vi "Set Line.vi"(8 "error in (no error)":errorcluster, 10 "First Visible Line":i32, 11 "ScintillaNET in":refnum<class "ScintillaNET.lvclass">) -> (0 "error out":errorcluster, 3 "ScintillaNET out":refnum<class "ScintillaNET.lvclass">)   [LabVIEW 2018, in "ScintillaNET.lvclass"]
uses:
  ScintillaNET.lvclass
  ScintillaNET.lvclass/ScintillaNET.ctl
  D:/project/hobby/LF2R/LabVIEW/source/ScintillaNET/dll/ScintillaNET.dll
  dll/ScintillaNET.dll
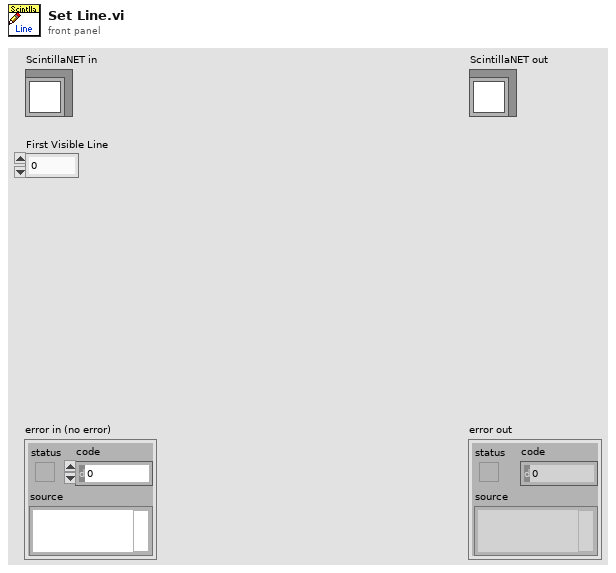
[diagram p1: front panel]
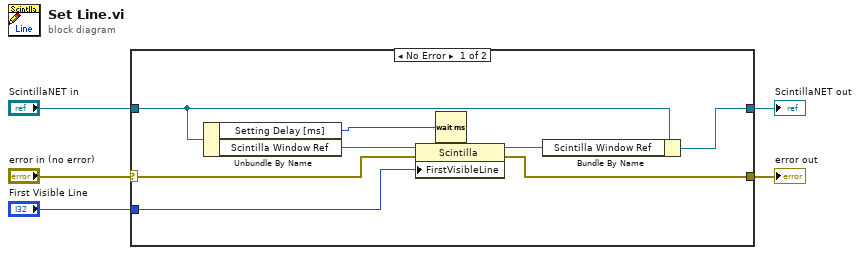
[diagram p0: block diagram]
diagram:
  n1 = case shown="No Error" "error in (no error)" {
    selector: "error in (no error)" -> [w11 w15]
    tunnel: [w9 w15] -> w4
    tunnel: [w8 w14] -> w2
    tunnel: "ScintillaNET in" -> [w13 w14]
    tunnel: "First Visible Line" -> [w10 _]
    frame No Error {
      n2 = Unbundle By Name(w13) -> ("Setting Delay [ms]"=w6:u32, "Scintilla Window Ref"=w12:refnum<k24>)
      n3 = property class="Scintilla"(reference=w12, error in=w11, "FirstVisibleLine"=w10) -> (reference out=w7:refnum<k24>, error out=w9:errorcluster)
      n4 = Wait (ms)(milliseconds to wait=w6) -> ()  [unwired: 1 out]
      n5 = Bundle By Name(cluster=w13, "Scintilla Window Ref"=w7) -> (w8:refnum<class "ScintillaNET.lvclass">)
    }
    frame Error {
    }
  }
  "error out" <- w4
  "ScintillaNET out" <- w2
